vi "FootPedalWait.vi"() -> ()   [LabVIEW 2022 SP3]
uses:
  <vilib>/Utility/inputDevices.llb/keyboardAcquire.vi
  <vilib>/Utility/inputDevices.llb/closeKeyboard.vi
panel:
  out "Stop?":bool
  out "Keys Pressed":T1(array[ring])
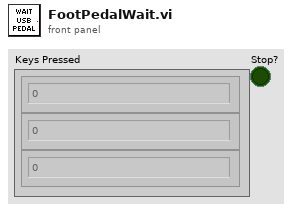
[diagram p1: front panel]
types:
  T1 = enum16{"0", "1", "2", "3", "4", "5", "6", "7", "8", "9", "A", "B", "C", "D", "E", "F", "G", "H", "I", "J", "K", "L", "M", "N", "O", "P", "Q", "R", "S", "T", "U", "V", "W", "X", "Y", "Z", "F1", "F2", "F3", "F4", "F5", "F6", "F7", "F8", "F9", "F10", "F11", "F12", "F13", "F14", "F15", "ADD", "BACK", "BACKSLASH", "CAPITAL", "COMMA", "DECIMAL", "DELETE", "DIVIDE", "DOWN", "END", "EQUALS", "ESCAPE", "GRAVE (`)", "HOME", "INSERT", "LBRACKET", "LCONTROL", "LEFT", "L ALT", "LSHIFT", "LWIN", "MINUS", "MULTIPLY", "NEXT", "NUMLOCK", "NUMPAD_0", "NUMPAD_1", "NUMPAD_2", "NUMPAD_3", "NUMPAD_4", "NUMPAD_5", "NUMPAD_6", "NUMPAD_7", "NUMPAD_8", "NUMPAD_9", "PAUSE", "PERIOD", "PRIOR (PG UP)", "RBRACKET", "RCONTROL", "RETURN", "RIGHT", "R ALT", "RSHIFT", "RWIN", "SCROLL", "SEMICOLON", "SLASH", "SPACE", "SUBTRACT", "TAB", "UP", "ENTER (num pad)", "' (quote)"}[]
  T2 = enum16{"0", "1", "2", "3", "4", "5", "6", "7", "8", "9", "A", "B", "C", "D", "E", "F", "G", "H", "I", "J", "K", "L", "M", "N", "O", "P", "Q", "R", "S", "T", "U", "V", "W", "X", "Y", "Z", "F1", "F2", "F3", "F4", "F5", "F6", "F7", "F8", "F9", "F10", "F11", "F12", "F13", "F14", "F15", "ADD", "BACK", "BACKSLASH", "CAPITAL", "COMMA", "DECIMAL", "DELETE", "DIVIDE", "DOWN", "END", "EQUALS", "ESCAPE", "GRAVE (`)", "HOME", "INSERT", "LBRACKET", "LCONTROL", "LEFT", "L ALT", "LSHIFT", "LWIN", "MINUS", "MULTIPLY", "NEXT", "NUMLOCK", "NUMPAD_0", "NUMPAD_1", "NUMPAD_2", "NUMPAD_3", "NUMPAD_4", "NUMPAD_5", "NUMPAD_6", "NUMPAD_7", "NUMPAD_8", "NUMPAD_9", "PAUSE", "PERIOD", "PRIOR (PG UP)", "RBRACKET", "RCONTROL", "RETURN", "RIGHT", "R ALT", "RSHIFT", "RWIN", "SCROLL", "SEMICOLON", "SLASH", "SPACE", "SUBTRACT", "TAB", "UP", "ENTER (num pad)", "' (quote)"}
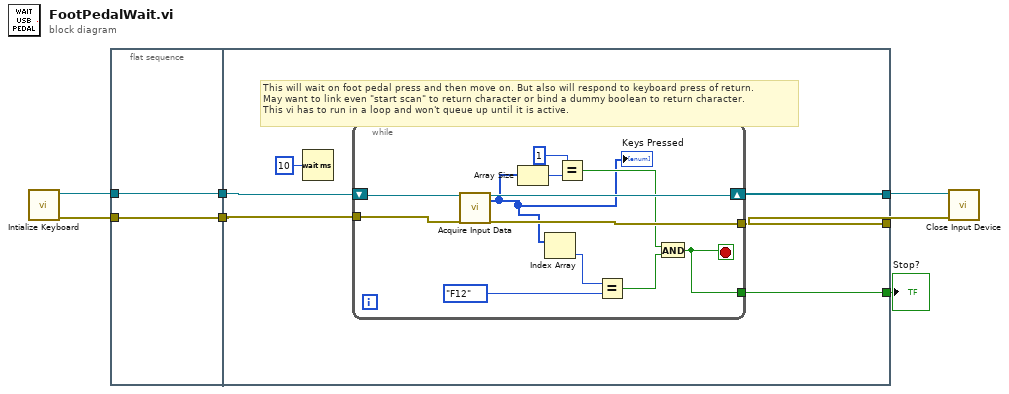
[diagram p0: block diagram]
diagram:
  n1 = call <vilib>:"Intialize Keyboard.vi"() -> ("error out"=w5:errorcluster, "device ID"=w7:refnum<k1>)  [unwired: 1 in, 9 out]
  n2 = flat-sequence {
    tunnel: w5 -> [w8]
    tunnel: w7 -> [w9]
    tunnel: [w9] -> w2
    tunnel: [w8] -> w1
    tunnel: [w14] -> w6
    tunnel: [w12] -> w4
    tunnel: [w11] -> w3
    tunnel: w2 -> [w15]
    tunnel: w1 -> [w13]
    frame #0 {
    }
    frame #1 {
      # "This will wait on foot pedal press and then move on. But also will respond to keyboard press of return.\nMay want to link even \"start scan\" to return character or bind a dummy boolean to return character.\nThis vi has to run in a loop and won't queue up until it is active."
      n3 = Wait (ms)(milliseconds to wait=u32 10) -> ()  [unwired: 1 out]
      n4 = while {
        shift-right: [w26] -> w14
        shift-left: w15 -> [w27]
        tunnel: w13 -> [w22]
        tunnel: [w21] -> w12
        tunnel: [w16] -> w11
        stop <- w16 stop-if-true
        n5 = call-poly <vilib>:"Acquire Input Data.vi"("device ID"=w27, "error in (no error)"=w22) -> ("device ID"=w26:refnum<k1>, "keys pressed"=w17:T1, "error out"=w21:errorcluster)  [unwired: 15 out]
        "Keys Pressed" <- w17
        n6 = Array Size(array=w17) -> (size(s)=w24:i32)
        n7 = Index Array(array=w17) -> (element=w19:T2)  [unwired: 1 in]
        n8 = Equal?(x=1, y=w24) -> (x = y?=w18:bool)
        n9 = Equal?(x=w19, y=T2."F12" ("Enum")) -> (x = y?=w20:bool)
        n10 = And(x=w18, y=w20) -> (x .and. y?=w16:bool)
      }
    }
  }
  n11 = call-poly <vilib>:"Close Input Device.vi"("error in (no error)"=w4, "device ID"=w6) -> ()  [unwired: 9 out]
  "Stop?" <- w3
